vi "Merge to Min MAx.vi"(10 "Rule":T1, 11 "Min Max":i32[][](array[numeric])) -> (2 "Rule Out":T1, 3 "Min Max":i32[][](array[numeric]))   [LabVIEW 2023]
uses:
  Cluster_Rule.ctl
  ENUM_Compare.ctl
  ENUM_Value Type.ctl
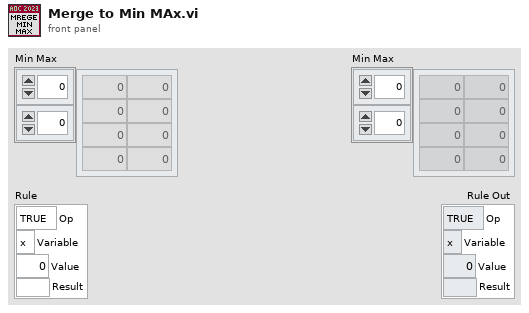
[diagram p1: front panel]
types:
  T1 = typedef "Cluster_Rule.ctl" = cluster{"Op":T2, "Variable":T3, "Value":i32, "Result":string}
  T2 = typedef "ENUM_Compare.ctl" = enum16{"TRUE", "<", ">", "<=", ">="}
  T3 = typedef "ENUM_Value Type.ctl" = enum16{"x", "m", "a", "s"}
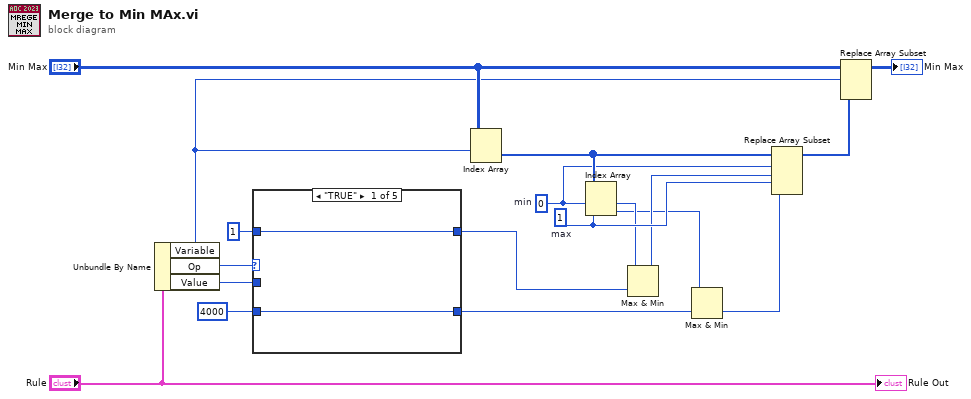
[diagram p0: block diagram]
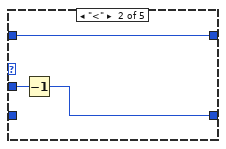
[diagram p2: hidden frame]
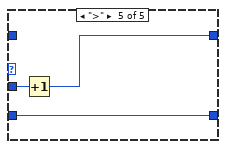
[diagram p5: hidden frame]
diagram:
  w12 = 1  # max
  w13 = 0  # min
  n1 = Unbundle By Name("Rule") -> ("Variable"=w15:T3, "Op"=w6:T2, "Value"=w1:i32)
  n2 = case shown="\"TRUE\"" w6 {
    tunnel: 1 ("y") -> [w20 w23 w25 _ _]
    tunnel: [w20 w23 w25 w27 w28] -> w4
    tunnel: 4000 ("y") -> [w19 _ _ w26 w29]
    tunnel: [w19 w21 w24 w26 w29] -> w2
    tunnel: w1 -> [_ w22 w24 w27 w30]
    frame "TRUE" {
    }
    frame "<" {
      n3 = Decrement(x=w22) -> (x-1=w21:i32)
    }
    frame "<=" {
    }
    frame ">=" {
    }
    frame ">" {
      n4 = Increment(x=w30) -> (x+1=w28:i32)
    }
  }
  n5 = Index Array(array="Min Max", index (row)=w15) -> (element=w18:i32[])  [unwired: 1 in]
  n6 = Index Array(array=w18, index #1=w13, index #2=w12) -> (element #1=w11:i32, element #2=w9:i32)
  n7 = Max & Min(x=w11, y=w4) -> (max(x,y)=w10:i32)  [unwired: 1 out]
  n8 = Max & Min(x=w9, y=w2) -> (min(x,y)=w8:i32)  [unwired: 1 out]
  n9 = Replace Array Subset(array=w18, new element #1=w10, index #1=w13, new element #2=w8, index #2=w12) -> (w14:i32[])
  n10 = Replace Array Subset(array="Min Max", new element=w14, index (row)=w15) -> (→"Min Max":i32[][])  [unwired: 1 in]
  "Rule Out" <- "Rule"
